vi "Find Custom Error.vi"(11 "VI References":refnum<vi>[](array[refnum])) -> (3 "Custom Errors":T1[](array[typedef]))   [LabVIEW 2021, in "TAF Proj Document Type.lvlib" / "Project Parser.lvlib"]
uses:
  <vilib>/Wovalab/AntiDoc/Document Type/Add-ons/LabVIEW TAF Project/Project Parser/Project Parser.lvlib
  <vilib>/Wovalab/AntiDoc/Document Type/Add-ons/LabVIEW TAF Project/Project Parser/Custom Error Info.ctl
  <vilib>/regexp/Match Regular Expression.xnode
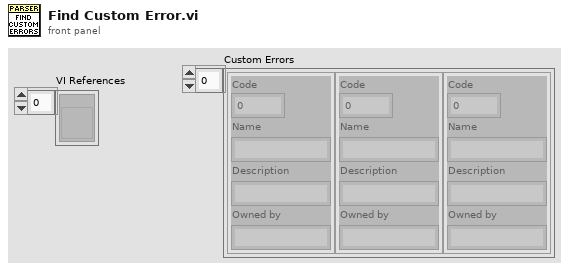
[diagram p1: front panel]
types:
  T1 = typedef "TAF Proj Document Type.lvlib/Project Parser.lvlib/Custom Error Info.ctl" = cluster{"Code":i32, "Name":string, "Description":string, "Owned by":string}
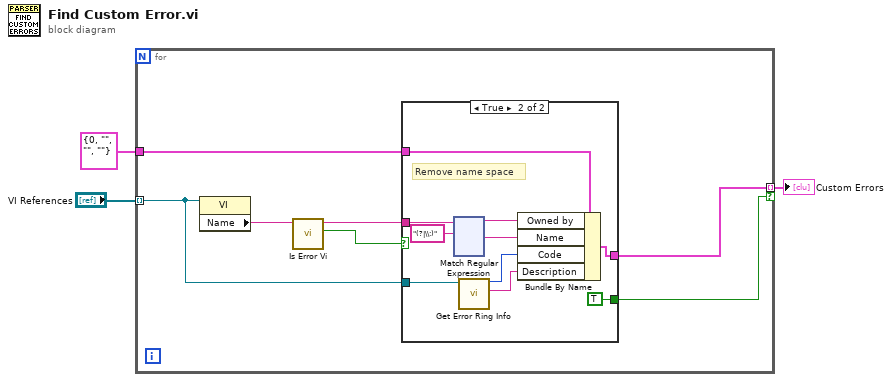
[diagram p0: block diagram]
diagram:
  n1 = for {
    tunnel: "VI References" -> [w4] mode=indexing
    tunnel: T1 {"Code"=0, "Name"="", "Description"="", "Owned by"=""} ("Custom Error Info") -> [w10]
    tunnel: [w9] -> w1 mode=indexing if=w5
    n2 = property class="VI"(reference=w4) -> ("Name"=w8:string)  [unwired: 1 in, 2 out]
    n3 = call <vilib>:"Is Error Vi.vi"("Vi Name"=w8) -> ("Error Vi?"=w6:bool, "Error Name"=w7:string)  [unwired: 9 in]
    n4 = case shown="True" w6 {
      tunnel: w7 -> [_ w13]
      tunnel: w10 -> [_ w18]
      tunnel: [_ w17] -> w9
      tunnel: [_ TRUE] -> w5
      tunnel: w4 -> [_ w15]
      frame False {
      }
      frame True {
        # "Remove name space"
        n5 = xnode "Match Regular Expression"("input string"=w13, "regular expression"="(?|\\:)") -> ("before match"=w11:string, "after match"=w12:string)  [unwired: 4 in, 3 out]
        n6 = call <vilib>:"Get Error Ring Info.vi"("Error VI Refnum"=w15) -> ("Custom Description"=w19:string, "code"=w20:i32)  [unwired: 8 in, 1 out]
        n7 = Bundle By Name(cluster=w18, "Owned by"=w11, "Name"=w12, "Code"=w20, "Description"=w19) -> (w17:T1)
      }
    }
  }
  "Custom Errors" <- w1
